vi "PhotonPoseEstimator_averageBestTargetsStrategy_calc.vi"(4 "TimeStamp":dbl, 5 "RobotToCamera":T3={"TRANSLATION3D"={"X"=0.0, "Y"=0.0, "Z"=0.0}, "ROTATION3D"={"Q_quaternion"={"R"=1.0, "V"=[0.0, 0.0, 0.0]}}, "XF"=FALSE} {"TRANSLATION3D"."Z" format="%14.3f"; "TRANSLATION3D"."Y" format="%14.3f"; "TRANSLATION3D"."X" format="%14.3f"}, 6 "FieldTargetPose":T7={"Translation3d"={"X"=0.0, "Y"=0.0, "Z"=0.0}, "Rotation3d"={"Q_quaternion"={"R"=1.0, "V"=[0.0, 0.0, 0.0]}}} {"Translation3d"."Z" format="%14.3f"; "Translation3d"."Y" format="%14.3f"; "Translation3d"."X" format="%14.3f"}, 7 "Target Ambiguity":dbl, 8 "In Total Inverse Amb":dbl, 9 "TransformToEvaluate":T3={"TRANSLATION3D"={"X"=0.0, "Y"=0.0, "Z"=0.0}, "ROTATION3D"={"Q_quaternion"={"R"=1.0, "V"=[0.0, 0.0, 0.0]}}, "XF"=FALSE} {"TRANSLATION3D"."Z" format="%14.3f"; "TRANSLATION3D"."Y" format="%14.3f"; "TRANSLATION3D"."X" format="%14.3f"}, 10 "Targets":T1[](array[typedef]) {"AltCameraToTarget"."TRANSLATION3D"."Z" format="%14.3f"; "AltCameraToTarget"."TRANSLATION3D"."Y" format="%14.3f"; "AltCameraToTarget"."TRANSLATION3D"."X" format="%14.3f"; "BestCameraToTarget"."TRANSLATION3D"."Z" format="%14.3f"; "BestCameraToTarget"."TRANSLATION3D"."Y" format="%14.3f"; "BestCameraToTarget"."TRANSLATION3D"."X" format="%14.3f"}, 11 "In Potential Robot Loc":T8[](array[typedef]) {"PhotonEstimatedRobotPose"."targetsUsed"."AltCameraToTarget"."TRANSLATION3D"."Z" format="%14.3f"; "PhotonEstimatedRobotPose"."targetsUsed"."AltCameraToTarget"."TRANSLATION3D"."Y" format="%14.3f"; "PhotonEstimatedRobotPose"."targetsUsed"."AltCameraToTarget"."TRANSLATION3D"."X" format="%14.3f"; "PhotonEstimatedRobotPose"."targetsUsed"."BestCameraToTarget"."TRANSLATION3D"."Z" format="%14.3f"; "PhotonEstimatedRobotPose"."targetsUsed"."BestCameraToTarget"."TRANSLATION3D"."Y" format="%14.3f"; "PhotonEstimatedRobotPose"."targetsUsed"."BestCameraToTarget"."TRANSLATION3D"."X" format="%14.3f"; "PhotonEstimatedRobotPose"."EstimatedPose"."Translation3d"."Z" format="%14.3f"; "PhotonEstimatedRobotPose"."EstimatedPose"."Translation3d"."Y" format="%14.3f"; "PhotonEstimatedRobotPose"."EstimatedPose"."Translation3d"."X" format="%14.3f"}) -> (0 "Out Total Inverse Amb":dbl, 3 "Out Potential Robot Loc":T8[](array[typedef]) {"PhotonEstimatedRobotPose"."targetsUsed"."AltCameraToTarget"."TRANSLATION3D"."Z" format="%14.3f"; "PhotonEstimatedRobotPose"."targetsUsed"."AltCameraToTarget"."TRANSLATION3D"."Y" format="%14.3f"; "PhotonEstimatedRobotPose"."targetsUsed"."AltCameraToTarget"."TRANSLATION3D"."X" format="%14.3f"; "PhotonEstimatedRobotPose"."targetsUsed"."BestCameraToTarget"."TRANSLATION3D"."Z" format="%14.3f"; "PhotonEstimatedRobotPose"."targetsUsed"."BestCameraToTarget"."TRANSLATION3D"."Y" format="%14.3f"; "PhotonEstimatedRobotPose"."targetsUsed"."BestCameraToTarget"."TRANSLATION3D"."X" format="%14.3f"; "PhotonEstimatedRobotPose"."EstimatedPose"."Translation3d"."Z" format="%14.3f"; "PhotonEstimatedRobotPose"."EstimatedPose"."Translation3d"."Y" format="%14.3f"; "PhotonEstimatedRobotPose"."EstimatedPose"."Translation3d"."X" format="%14.3f"})   [LabVIEW 2019, in "PhotonVisionLib.lvlib"]
doc: "This is an internal function. Use Update or Update_Pipeline instead of this function.\n\nDetermine the best target based the weighted average position of valid potential positions."
uses:
  PhotonVisionLib.lvlib
  TypeDef/PhotonPoseEstimator_PotentialRobotLocation.ctl
  TypeDef/PhotonEstimatedRobotPoseType.ctl
  <vilib>/Rock Robotics/WPI/ThirdParty/JAS_Junk/TrajLib/TypeDef/POSE3D.ctl
  <vilib>/Rock Robotics/WPI/ThirdParty/JAS_Junk/TrajLib/TypeDef/TRANSLATION3D.ctl
  <vilib>/Rock Robotics/WPI/ThirdParty/JAS_Junk/TrajLib/TypeDef/ROTATION3D.ctl
  <vilib>/Rock Robotics/WPI/ThirdParty/JAS_Junk/TrajLib/TypeDef/QUATERNION.ctl
  TypeDef/PhotonTrackedTargetType.ctl
  TypeDef/TargetCornerType.ctl
  <vilib>/Rock Robotics/WPI/ThirdParty/JAS_Junk/TrajLib/TypeDef/TRANSFORM3D.ctl
  Enum/PhotonPoseStrategy_ENUM.ctl
  <vilib>/Rock Robotics/WPI/ThirdParty/JAS_Junk/TrajLib/VI/Pose3d_getTranslation3d.vi
  <vilib>/Rock Robotics/WPI/ThirdParty/JAS_Junk/TrajLib/VI/Pose3d_getRotation3d.vi
  <vilib>/Rock Robotics/WPI/ThirdParty/JAS_Junk/TrajLib/VI/Transform3d_GetTranslation3d.vi
  <vilib>/Rock Robotics/WPI/ThirdParty/JAS_Junk/TrajLib/VI/Transform3d_GetRotation3d.vi
  <vilib>/Rock Robotics/WPI/ThirdParty/JAS_Junk/TrajLib/VI/Translation3d_Plus.vi
  <vilib>/Rock Robotics/WPI/ThirdParty/JAS_Junk/TrajLib/VI/Translation3d_RotateBy.vi
  <vilib>/Rock Robotics/WPI/ThirdParty/JAS_Junk/TrajLib/VI/Pose3d_New_Trans3dRot3d.vi
  <vilib>/Rock Robotics/WPI/ThirdParty/JAS_Junk/TrajLib/VI/Rotation3d_Plus.vi
  <vilib>/Rock Robotics/WPI/ThirdParty/JAS_Junk/TrajLib/VI/Transform3d_Create_Trans3dRot3d.vi
  <vilib>/Rock Robotics/WPI/ThirdParty/JAS_Junk/TrajLib/VI/Rotation3d_UnaryMinus.vi
  <vilib>/Rock Robotics/WPI/ThirdParty/JAS_Junk/TrajLib/VI/Translation3d_UnaryMinus.vi
  <vilib>/Rock Robotics/WPI/ThirdParty/JAS_Junk/TrajLib/VI/Translation3d_Create.vi
  <vilib>/Rock Robotics/WPI/ThirdParty/JAS_Junk/TrajLib/VI/Rotation3d_GetQuaterion.vi
  <vilib>/Rock Robotics/WPI/ThirdParty/JAS_Junk/TrajLib/VI/Quaternion_New.vi
  <vilib>/Rock Robotics/WPI/ThirdParty/JAS_Junk/TrajLib/VI/Quaternion_Times.vi
  <vilib>/Rock Robotics/WPI/ThirdParty/JAS_Junk/TrajLib/VI/Quaternion_Inverse.vi
  <vilib>/Rock Robotics/WPI/ThirdParty/JAS_Junk/TrajLib/VI/Quaternion_Get_All.vi
  <vilib>/Rock Robotics/WPI/ThirdParty/JAS_Junk/TrajLib/VI/Rotation3d_RotateBy.vi
  <vilib>/Rock Robotics/WPI/ThirdParty/JAS_Junk/TrajLib/VI/Rotation3d_Create_Quaternion.vi
  <vilib>/Rock Robotics/WPI/ThirdParty/JAS_Junk/TrajLib/VI/Quaternion_Normalize.vi
  <vilib>/Rock Robotics/WPI/ThirdParty/JAS_Junk/TrajLib/VI/Quaternion_New_Default.vi
  <vilib>/Rock Robotics/WPI/ThirdParty/JAS_Junk/TrajLib/Trajectory_Library.lvlib
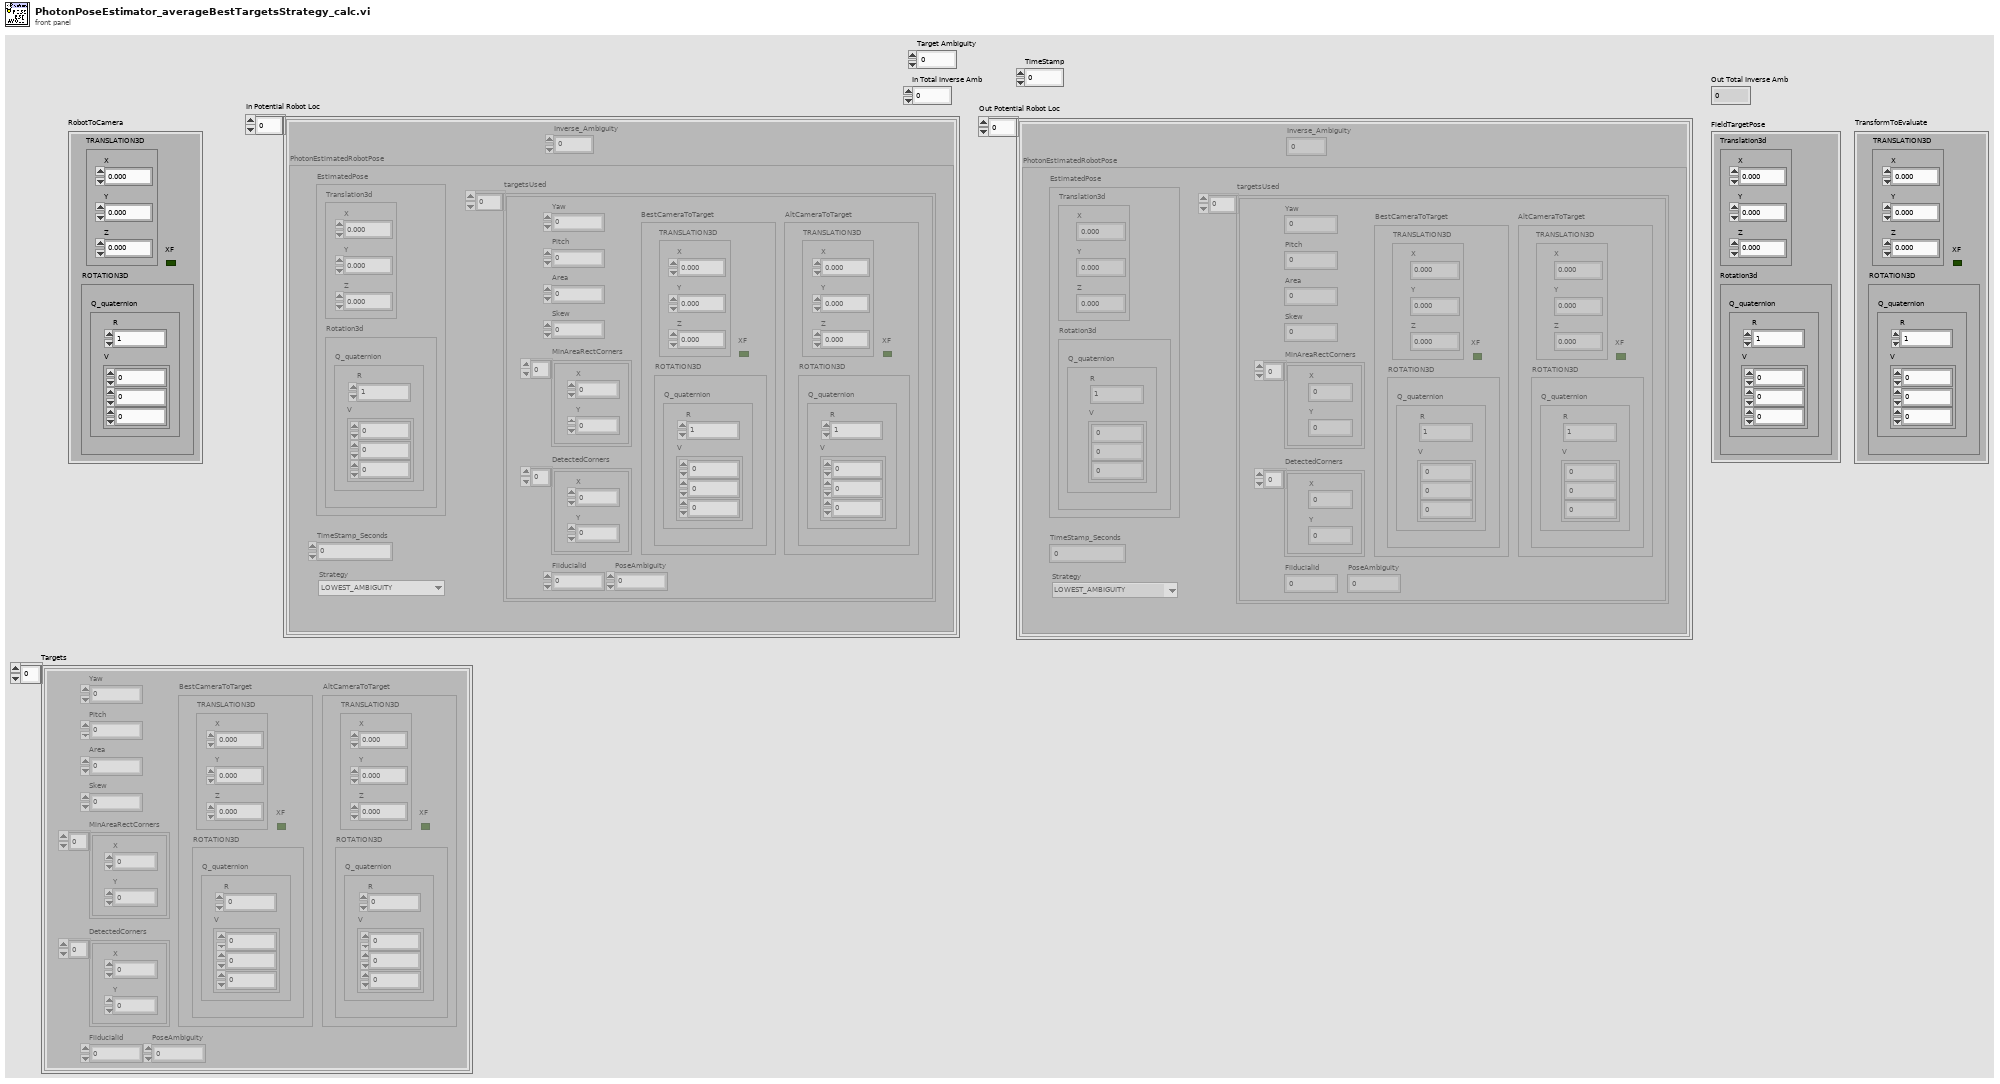
[diagram p1: front panel]
types:
  T1 = typedef "PhotonVisionLib.lvlib/PhotonTrackedTargetType.ctl" = cluster{"Yaw":dbl, "Pitch":dbl, "Area":dbl, "Skew":dbl, "MinAreaRectCorners":T2[], "BestCameraToTarget":T3, "FiiducialId":i32, "AltCameraToTarget":T3, "PoseAmbiguity":dbl, "DetectedCorners":T2[]}
  T2 = typedef "PhotonVisionLib.lvlib/TargetCornerType.ctl" = cluster{"X":dbl, "Y":dbl}
  T3 = typedef "Trajectory_Library.lvlib/TRANSFORM3D.ctl" = cluster{"TRANSLATION3D":T4, "ROTATION3D":T5, "XF":bool}
  T4 = typedef "Trajectory_Library.lvlib/TRANSLATION3D.ctl" = cluster{"X":dbl, "Y":dbl, "Z":dbl}
  T5 = typedef "Trajectory_Library.lvlib/ROTATION3D.ctl" = cluster{"Q_quaternion":T6}
  T6 = typedef "Trajectory_Library.lvlib/QUATERNION.ctl" = cluster{"R":dbl, "V":dbl[]}
  T7 = typedef "Trajectory_Library.lvlib/POSE3D.ctl" = cluster{"Translation3d":T4, "Rotation3d":T5}
  T8 = typedef "PhotonVisionLib.lvlib/PhotonPoseEstimator_PotentialRobotLocation.ctl" = cluster{"Inverse_Ambiguity":dbl, "PhotonEstimatedRobotPose":T9}
  T9 = typedef "PhotonVisionLib.lvlib/PhotonEstimatedRobotPoseType.ctl" = cluster{"EstimatedPose":T7, "TimeStamp_Seconds":dbl, "targetsUsed":T1[], "Strategy":T10}
  T10 = typedef "PhotonVisionLib.lvlib/PhotonPoseStrategy_ENUM.ctl" = enum16{"LOWEST_AMBIGUITY", "CLOSEST_TO_CAMERA_HEIGHT", "CLOSEST_TO_REFERENCE_POSE", "CLOSEST_TO_LAST_POSE", "AVERAGE_BEST_TARGETS", "MULTI_TAG_PNP_ON_COPROCESSOR", "MULTI_TAG_PNP_ON_RIO"}
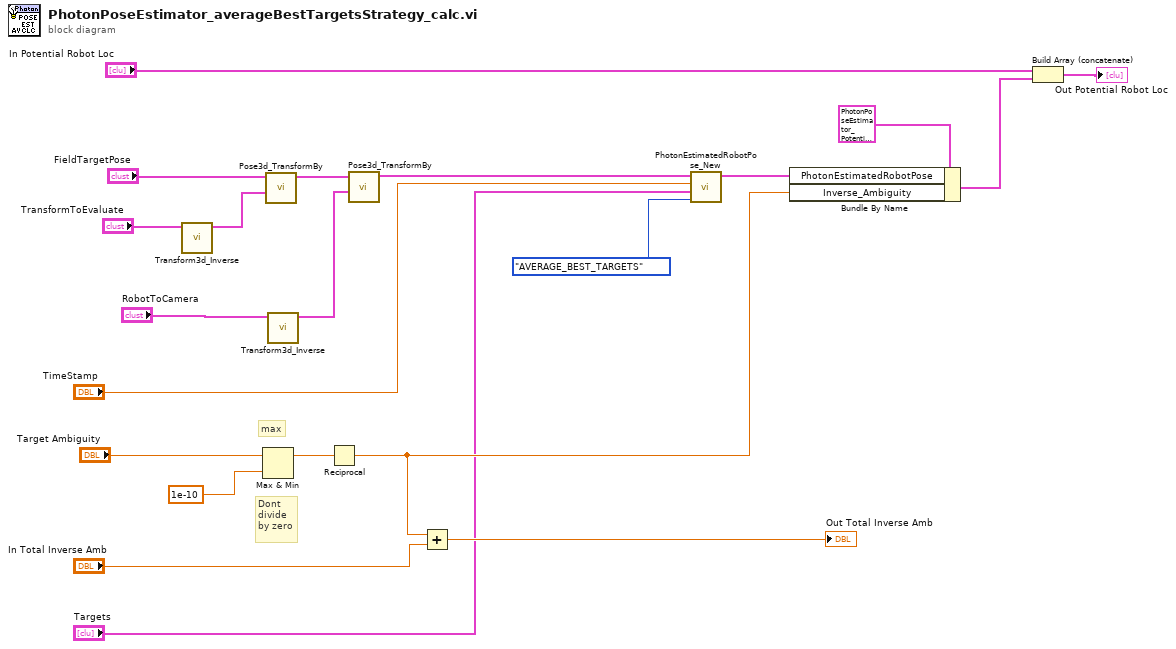
[diagram p0: block diagram]
diagram:
  # "Dont\ndivide\nby zero"
  # "max"
  n1 = call <vilib>:"Transform3d_Inverse.vi"("inTransform3d"="TransformToEvaluate") -> ("outTransform3d"=w20:T3)  [unwired: 10 in]
  n2 = Max & Min(x="Target Ambiguity", y=1e-10) -> (max(x,y)=w8:dbl)  [unwired: 1 out]
  n3 = call <vilib>:"Pose3d_TransformBy.vi"("other Transform3d"=w20, "in Pose3d"="FieldTargetPose") -> ("out POSE3d"=w16:T7)  [unwired: 9 in]
  n4 = call <vilib>:"Transform3d_Inverse.vi"("inTransform3d"="RobotToCamera") -> ("outTransform3d"=w18:T3)  [unwired: 10 in]
  n5 = Reciprocal(x=w8) -> (1/x=w6:dbl)
  n6 = call <vilib>:"Pose3d_TransformBy.vi"("other Transform3d"=w18, "in Pose3d"=w16) -> ("out POSE3d"=w17:T7)  [unwired: 9 in]
  n7 = Add(x=w6, y="In Total Inverse Amb") -> (x+y=→"Out Total Inverse Amb":dbl)
  n8 = call "PhotonEstimatedRobotPose_New.vi"("Strategy"=PhotonPoseStrategy_ENUM."AVERAGE_BEST_TARGETS", "targetsUsed"="Targets", "TimeStamp_Seconds"="TimeStamp", "EstimatedPose"=w17) -> ("PhotonEstimatedRobotPose"=w14:T9)  [unwired: 7 in]
  n9 = Bundle By Name(cluster=T8 {"Inverse_Ambiguity"=0.0, "PhotonEstimatedRobotPose"={"EstimatedPose"={"Translation3d"={"X"=0.0, "Y"=0.0, "Z"=0.0}, "Rotation3d"={"Q_quaternion"={"R"=1.0, "V"=[0.0, 0.0, 0.0]}}}, "TimeStamp_Seconds"=0.0, "targetsUsed"=[], "Strategy"=enum."LOWEST_AMBIGUITY"}} ("PotentialRobotLocation"), "PhotonEstimatedRobotPose"=w14, "Inverse_Ambiguity"=w6) -> (w11:T8)
  n10 = Build Array (concatenate)("In Potential Robot Loc", w11) -> (→"Out Potential Robot Loc":T8[])
